vi "Check for Missing Modules.vi"(8 "error in (no error)":errorcluster, 11 "SystemConfigRepo in":refnum<class "SystemConfigRepo.lvclass">) -> (0 "error out":errorcluster, 2 "Missing Module?":bool)   [LabVIEW 2014, in "PL Framework Configuration Tool.lvlib" / "SystemConfigRepo.lvclass"]
uses:
  SystemConfigRepo.lvclass
  Missing Plugin/module/configuration/Missing Plugin configuration.lvclass
  <vilib>/NI/Configuration Framework/serializable configuration/NISE_CEF_serializable configuration.lvclass
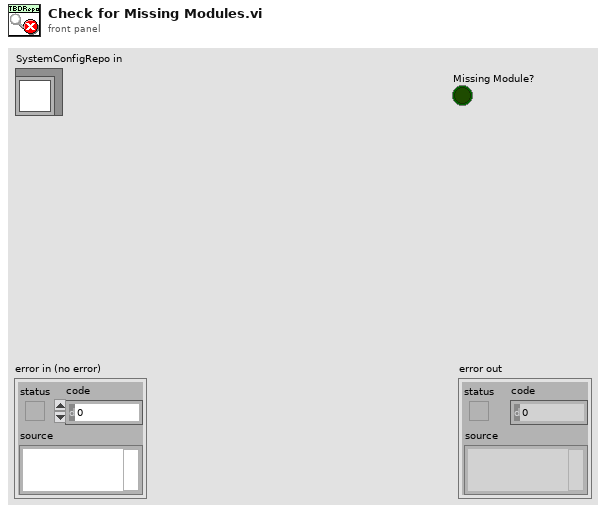
[diagram p1: front panel]
types:
  T1 = typedef "NISE_CEF_TreeSerializer.lvlib/memory hierarchy.ctl" = cluster{"hierarchy structure":T2, "instance data":refnum<class "NISE_CEF_serializable configuration.lvclass">[]}
  T2 = typedef "NISE_CEF_TreeSerializer.lvlib/full hierarchy.ctl" = cluster{"root":string, "hierarchy":T3[]}
  T3 = typedef "NISE_CEF_TreeSerializer.lvlib/hierarchy element.ctl" = cluster{"current node":string, "children":string[]}
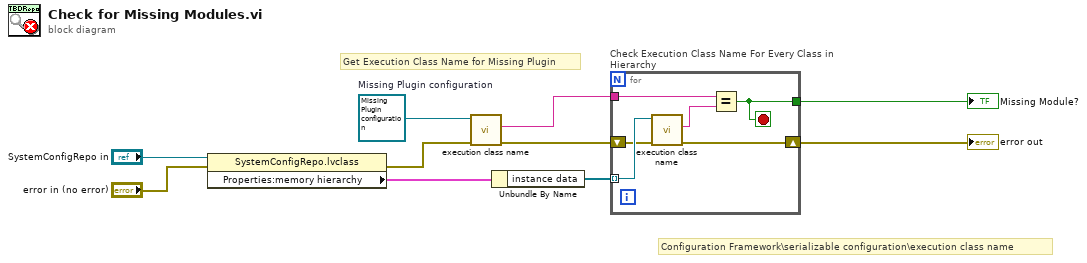
[diagram p0: block diagram]
diagram:
  w2 = refnum<class "Missing Plugin configuration.lvclass"> refnum  # Missing Plugin configuration
  # "Configuration Framework\\serializable configuration\\execution class name"
  # "Get Execution Class Name for Missing Plugin"
  n1 = property class="SystemConfigRepo.lvclass"(reference="SystemConfigRepo in", error in="error in (no error)") -> (error out=w4:errorcluster, "Properties:memory hierarchy"=w8:T1)  [unwired: 1 out]
  n2 = call-dynamic "execution class name.vi"("error in"=w4, "Missing Plugin configuration in"=w2) -> ("error out"=w3:errorcluster, "class name"=w1:string)  [unwired: 7 in, 1 out]
  n3 = Unbundle By Name(w8) -> ("instance data"=w7:refnum<class "NISE_CEF_serializable configuration.lvclass">[])
  n4 = for "Check Execution Class Name For Every Class in Hierarchy" {
    tunnel: w7 -> [w16] mode=indexing
    tunnel: w1 -> [w12]
    shift-right: [w14] -> w6
    shift-left: w3 -> [w15]
    tunnel: [w11] -> w5
    stop <- w11 stop-if-true
    n5 = call-dynamic "execution class name.vi"("error in"=w15, "configuration in"=w16) -> ("error out"=w14:errorcluster, "execution class"=w13:string)  [unwired: 7 in, 1 out]
    n6 = Equal?(x=w12, y=w13) -> (x = y?=w11:bool)
  }
  "error out" <- w6
  "Missing Module?" <- w5
